vi "svc_Input Array to Histogram Bin Configuration.vi"(7 "input data":dbl[](array[numeric]), 10 "range in":cluster{"minimum":dbl, "maximum":dbl}={"minimum"=-10.0, "maximum"=10.0}, 11 "number of bins in":i32=20) -> (2 "range out":cluster{"minimum":dbl, "maximum":dbl}={"minimum"=-10.0, "maximum"=10.0}, 3 "number of bins out":i32)   [LabVIEW 2017]
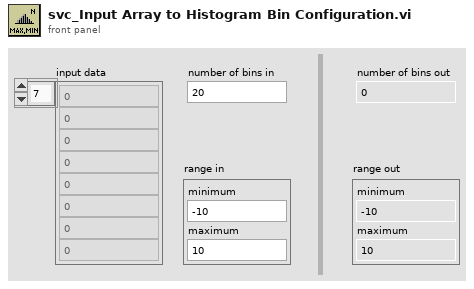
[diagram p1: front panel]
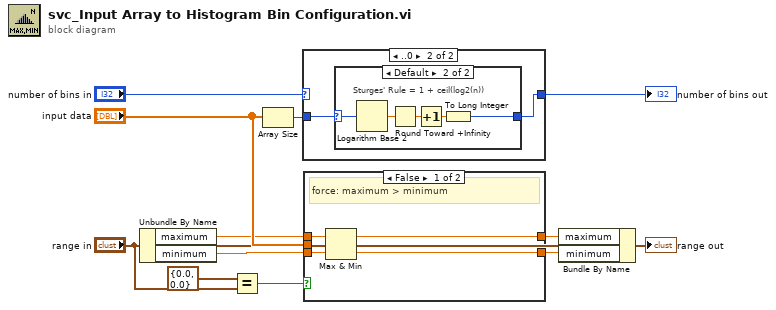
[diagram p0: block diagram]
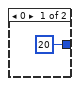
[diagram p3: hidden frame]
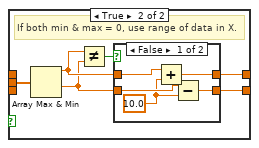
[diagram p4: hidden frame]
diagram:
  n1 = Unbundle By Name("range in") -> ("maximum"=w7:dbl, "minimum"=w8:dbl)
  n2 = Equal?(x=cluster{"minimum":dbl, "maximum":dbl} {"minimum"=0.0, "maximum"=0.0} ("range in"), y="range in") -> (x = y?=w3:bool)
  n3 = Array Size(array="input data") -> (size(s)=w10:i32)
  n4 = case shown="..0" "number of bins in" {
    selector: "number of bins in" -> [w13 _]
    tunnel: [w13 w15] -> w12
    tunnel: w10 -> [_ w14]
    frame 1, Default {
    }
    frame ..0 {
      n5 = case shown="Default" w14 {
        selector: w14 -> [_ w20]
        tunnel: [20 w21] -> w15
        frame 0 {
        }
        frame Default {
          # "Sturges' Rule = 1 + ceil(log2(n))"
          n6 = Logarithm Base 2(1:w20) -> (0:w19:dbl)
          n7 = Round Toward +Infinity(x=w19) -> (ceil(x): smallest int >= x=w18:dbl)
          n8 = Increment(x=w18) -> (x+1=w17:dbl)
          n9 = To Long Integer(number=w17) -> (32bit integer=w21:i32)
        }
      }
    }
  }
  "number of bins out" <- w12
  n10 = case shown="False" w3 {
    tunnel: "input data" -> [_ w31]
    tunnel: [w24 w29] -> w5
    tunnel: [w22 w27] -> w6
    tunnel: w7 -> [w25 _]
    tunnel: w8 -> [w23 _]
    frame False {
      # "force: maximum > minimum"
      n11 = Max & Min(x=w25, y=w23) -> (max(x,y)=w24:dbl, min(x,y)=w22:dbl)
    }
    frame True {
      # "If both min & max = 0, use range of data in X."
      n12 = Array Max & Min(array=w31) -> (max value=w28:dbl, min value=w26:dbl)  [unwired: 2 out]
      n13 = Not Equal?(x=w28, y=w26) -> (x != y?=w30:bool)
      n14 = case shown="False" w30 {
        tunnel: [w35 w38] -> w29
        tunnel: w28 -> [w36 w38]
        tunnel: [w33 w37] -> w27
        tunnel: w26 -> [w34 w37]
        frame False {
          w32 = 10.0 ("y")
          n15 = Add(x=w36, y=w32) -> (x+y=w35:dbl)
          n16 = Subtract(x=w34, y=w32) -> (x-y=w33:dbl)
        }
        frame True {
        }
      }
    }
  }
  n17 = Bundle By Name(cluster="range in", "maximum"=w5, "minimum"=w6) -> (→"range out":cluster{"minimum":dbl, "maximum":dbl})
